vi "Fill.vi"(8 "error in (no error)":errorcluster, 10 "Color":refnum<class "Color.lvclass">, 11 "Image in":refnum<class "Image.lvclass">) -> (0 "error out":errorcluster, 3 "Image out":refnum<class "Image.lvclass">)   [LabVIEW 2020, in "RPI.SenseHat.Display.lvlib" / "Image.lvclass"]
doc: "Fills the image of the given color."
uses:
  Image.lvclass
  Pixel/Pixel.lvclass
  Color/Color.lvclass
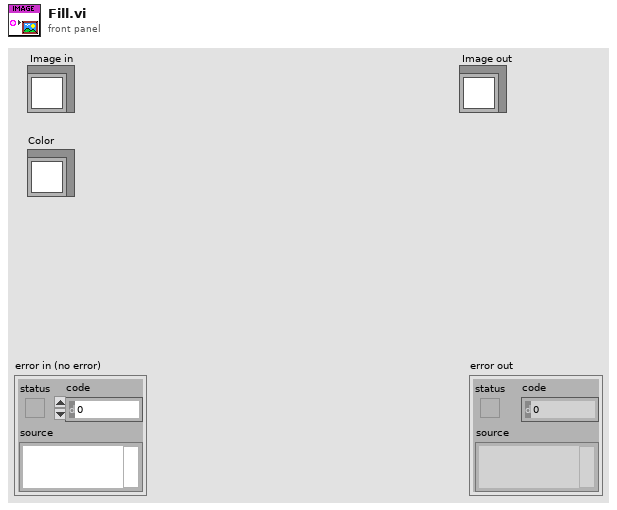
[diagram p1: front panel]
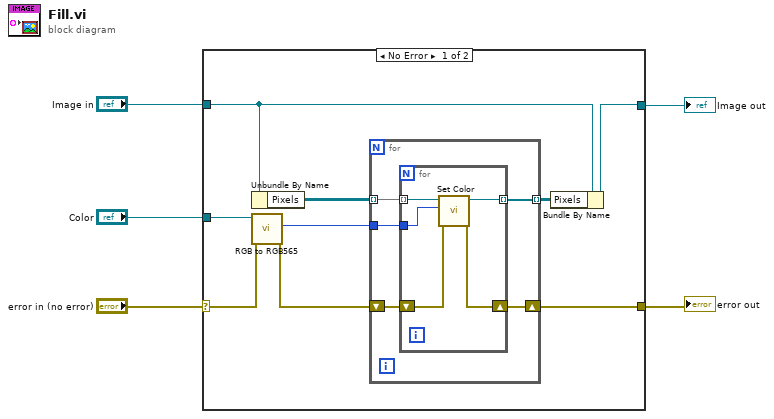
[diagram p0: block diagram]
diagram:
  n1 = case shown="No Error" "error in (no error)" {
    selector: "error in (no error)" -> [w6 w26]
    tunnel: [w12 w26] -> w4
    tunnel: [w11 w25] -> w2
    tunnel: "Image in" -> [w14 w25]
    tunnel: "Color" -> [w9 _]
    frame No Error {
      n2 = Unbundle By Name(w14) -> ("Pixels"=w13:refnum<class "Pixel.lvclass">[][])
      n3 = call "RGB to RGB565.vi"("error in (no error)"=w6, "Color in"=w9) -> ("error out"=w7:errorcluster, "Color"=w8:u16)  [unwired: 7 in, 1 out]
      n4 = for {
        tunnel: w13 -> [w19] mode=indexing
        shift-right: [w18] -> w12
        shift-left: w7 -> [w17]
        tunnel: [w16] -> w10 mode=indexing
        tunnel: w8 -> [w15]
        n5 = for {
          tunnel: w19 -> [w24] mode=indexing
          shift-right: [w23] -> w18
          shift-left: w17 -> [w22]
          tunnel: [w21] -> w16 mode=indexing
          tunnel: w15 -> [w20]
          n6 = call-dynamic "Set Color.vi"("error in (no error)"=w22, "Color"=w20, "Pixel in"=w24) -> ("error out"=w23:errorcluster, "Pixel out"=w21:refnum<class "Pixel.lvclass">)  [unwired: 7 in]
        }
      }
      n7 = Bundle By Name(cluster=w14, "Pixels"=w10) -> (w11:refnum<class "Image.lvclass">)
    }
    frame Error {
    }
  }
  "error out" <- w4
  "Image out" <- w2
